vi "TDT-Init RPcoX.vi"(0 "Output":T1, 7 "RPfilename":string, 9 "Sampling rate (Hz)":dbl format="%#_13g", 11 "error in (no error)":errorcluster) -> (4 "RPcoX":refnum<k7>, 15 "error out":errorcluster)   [LabVIEW 2020]
uses:
  Typedefs/TDT-Output source.ctl
  Typedefs/TDT-Device ID.ctl
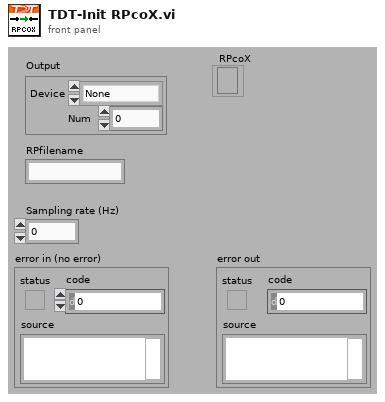
[diagram p1: front panel]
types:
  T1 = typedef "TDT-Output source.ctl" = cluster{"Device":T2, "Num":i32}
  T2 = typedef "TDT-Device ID.ctl" = enum16{"None", "PA5", "RP2", "RL2", "RA16", "RV8", "RX5", "RX6", "RX7", "RX8", "RZ2", "RZ5", "RZ6"}
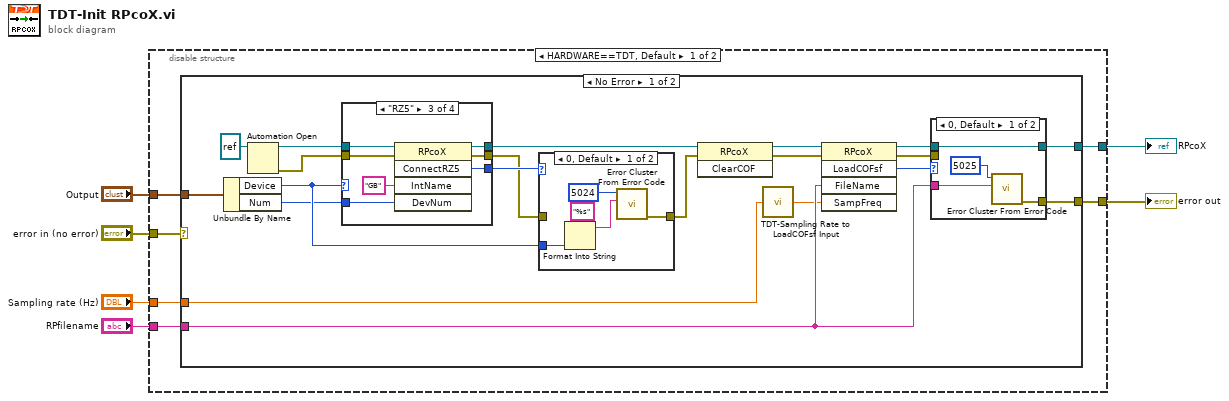
[diagram p0: block diagram]
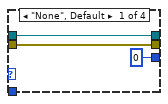
[diagram p3: hidden frame]
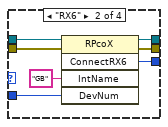
[diagram p4: hidden frame]
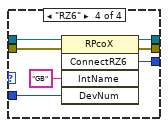
[diagram p5: hidden frame]
diagram:
  n1 = disable-structure shown="HARDWARE==TDT, Default" {
    disable-tunnel: [w11 _] -> w6
    disable-tunnel: "error in (no error)" -> [w9 w70]
    disable-tunnel: [w12 w70] -> w4
    disable-tunnel: "Output" -> [w10 _]
    disable-tunnel: "Sampling rate (Hz)" -> [w8 _]
    disable-tunnel: "RPfilename" -> [w7 _]
    frame condition #0 (active) {
      n2 = case shown="No Error" w9 {
        selector: w9 -> [_ w69]
        tunnel: [w19 w69] -> w12
        tunnel: [w20 _] -> w11
        tunnel: w10 -> [w27 _]
        tunnel: w8 -> [w22 _]
        tunnel: w7 -> [w21 _]
        frame No Error {
          n3 = Unbundle By Name(w27) -> ("Device"=w26:T2, "Num"=w25:i32)
          n4 = Automation Open(Automation Refnum=refnum<k7> refnum ("RPCOXLib.RPcoX")) -> (Automation Refnum=w31:refnum<k7>, error out=w30:errorcluster)  [unwired: 3 in]
          n5 = case shown="\"RZ5\"" w26 {
            tunnel: w31 -> [w40 w48 w55 w62]
            tunnel: w30 -> [w41 w46 w53 w60]
            tunnel: [0 ("ConnectRX6") w45 w52 w59] -> w29
            tunnel: [w41 w44 w51 w58] -> w28
            tunnel: [w40 w43 w50 w57] -> w24
            tunnel: w25 -> [_ w42 w49 w56]
            frame "None", Default {
            }
            frame "RX6" {
              n6 = invoke class="RPcoX" method="ConnectRX6"(reference=w48, error in=w46, "IntName"="GB", "DevNum"=w42) -> (reference out=w43:refnum<k7>, error out=w44:errorcluster, "ConnectRX6"=w45:i32)  [unwired: 1 in, 2 out]
            }
            frame "RZ5" {
              n7 = invoke class="RPcoX" method="ConnectRZ5"(reference=w55, error in=w53, "IntName"="GB", "DevNum"=w49) -> (reference out=w50:refnum<k7>, error out=w51:errorcluster, "ConnectRZ5"=w52:i32)  [unwired: 1 in, 2 out]
            }
            frame "RZ6" {
              n8 = invoke class="RPcoX" method="ConnectRZ6"(reference=w62, error in=w60, "IntName"="GB", "DevNum"=w56) -> (reference out=w57:refnum<k7>, error out=w58:errorcluster, "ConnectRZ6"=w59:i32)  [unwired: 1 in, 2 out]
            }
          }
          n9 = case shown="0, Default" w29 {
            tunnel: w28 -> [_ w68]
            tunnel: [w66 w68] -> w23
            tunnel: w26 -> [w65 _]
            frame 0, Default {
              n10 = Format Into String(format string="%s", w65) -> (resulting string=w64:string)  [unwired: 2 in, 1 out]
              n11 = call <vilib>:"Error Cluster From Error Code.vi"("error message (\"\")"=w64, "error code (0)"=5024) -> ("error out"=w66:errorcluster)  [unwired: 7 in]
            }
            frame 1 {
            }
          }
          n12 = invoke class="RPcoX" method="ClearCOF"(reference=w24, error in=w23) -> (reference out=w15:refnum<k7>, error out=w14:errorcluster)  [unwired: 1 in, 1 out]
          n13 = call "TDT-Sampling Rate to LoadCOFsf Input.vi"("Sampling rate (Hz)"=w22) -> ("LoadCOFsf Input"=w13:dbl)  [unwired: 14 in]
          n14 = invoke class="RPcoX" method="LoadCOFsf"(reference=w15, error in=w14, "FileName"=w21, "SampFreq"=w13) -> (reference out=w17:refnum<k7>, error out=w16:errorcluster, "LoadCOFsf"=w18:i32)  [unwired: 1 in, 2 out]
          n15 = case shown="0, Default" w18 {
            tunnel: w21 -> [w35 _]
            tunnel: w17 -> [w36 w38]
            tunnel: w16 -> [_ w37]
            tunnel: [w36 w38] -> w20
            tunnel: [w33 w37] -> w19
            frame 0, Default {
              n16 = call <vilib>:"Error Cluster From Error Code.vi"("error message (\"\")"=w35, "error code (0)"=5025) -> ("error out"=w33:errorcluster)  [unwired: 7 in]
            }
            frame 1 {
            }
          }
        }
        frame Error {
        }
      }
    }
    frame condition #1 {
    }
  }
  "error out" <- w4
  "RPcoX" <- w6
